vi "Compute P(x).vi"(6 "timeout (1000 ms)":i32=1000, 8 "error in (no error)":errorcluster, 10 "x":dbl, 11 "PolyA in":refnum<class "PolyA.lvclass">) -> (0 "error out":errorcluster, 2 "P(x)":dbl, 3 "PolyA out":refnum<class "PolyA.lvclass">, 4 "timed out?":bool)   [LabVIEW 2014, in "PolyA.lvclass"]
doc: "For polynomial coefficients = [a, b, c]\nP(x) = a + b*(x^1) + c*(x^2)"
uses:
  PolyA.lvclass
  Query Payload -- cluster.ctl
  PolyA.lvclass/PolyA.ctl
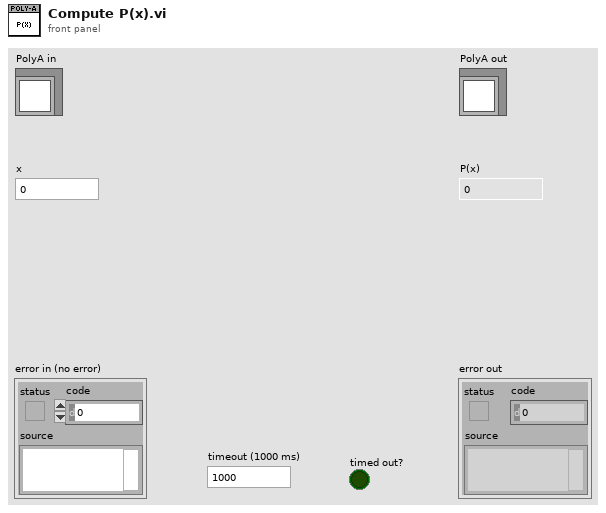
[diagram p1: front panel]
types:
  T1 = typedef "PolyA.lvclass/Query Payload -- cluster.ctl" = cluster{"value":dbl, "notifier":refnum<notifier>}
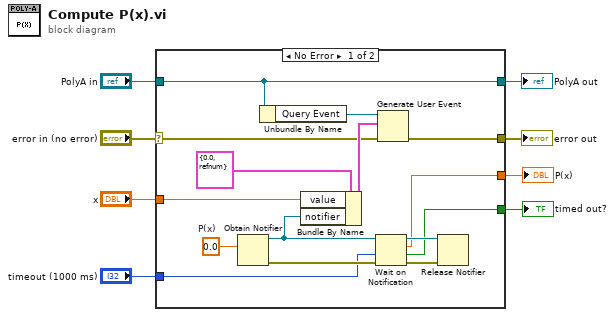
[diagram p0: block diagram]
diagram:
  n1 = case shown="No Error" "error in (no error)" {
    selector: "error in (no error)" -> [w11 w25]
    tunnel: [w10 w25] -> w7
    tunnel: [w17 w24] -> w5
    tunnel: "PolyA in" -> [w17 w24]
    tunnel: "timeout (1000 ms)" -> [w21 _]
    tunnel: [w18 _] -> w3
    tunnel: "x" -> [w14 _]
    tunnel: [w9 _] -> w1
    frame No Error {
      w23 = 0.0  # P(x)
      n2 = Obtain Notifier(notification data type=w23) -> (notifier out=w13:refnum<notifier>, error out=w22:errorcluster)  [unwired: 3 in, 1 out]
      n3 = Unbundle By Name(w17) -> ("Query Event"=w16:refnum<user-event>)
      n4 = Bundle By Name(cluster=T1 {"value"=0.0, "notifier"=refnum} ("Query Payload"), "value"=w14, "notifier"=w13) -> (w12:T1)
      n5 = Wait on Notification(notifier=w13, timeout in ms (-1)=w21, error in (no error)=w22) -> (notifier out=w20:refnum<notifier>, notification=w18:dbl, timed out?=w9:bool, error out=w19:errorcluster)  [unwired: 1 in]
      n6 = Generate User Event(user event=w16, event data cluster=w12, error in=w11) -> (error out=w10:errorcluster)  [unwired: 1 in, 1 out]
      n7 = Release Notifier(notifier=w20, error in (no error)=w19) -> ()  [unwired: 1 in, 3 out]
    }
    frame Error {
    }
  }
  "error out" <- w7
  "PolyA out" <- w5
  "P(x)" <- w3
  "timed out?" <- w1
